vi "RS232 Read Integer Curve Name Replace.vi"(8 "Hardware in":string, 9 "Step Setup in":string, 10 "Setup in":T1={"No.VI"=0, "Category"="", "StepName"="", "Seq setup flattened"="", "Comment"="", "Steps config."=[], "Jump config"=[], "Start"=0.0, "Increment"=0.0, "Name"="Pa", "Unit"="Pa", "Y data"=1, "Y prefix"="", "Y dB ref"=1.0, "Y unit"="", "Repeat State Array"=[]} {"Repeat State Array"."Start" format="%#_5g"; "Y dB ref" format="%.1f"; "Y data" items=["dB", "Lin"]; "Start" format="%#_5g"}, 11 "Type In":string) -> (3 "Inserted Names Out":string[](array[string]))   [LabVIEW 2013]
uses:
  CRYCustom and Run Seq.llb/CRYStep.ctl
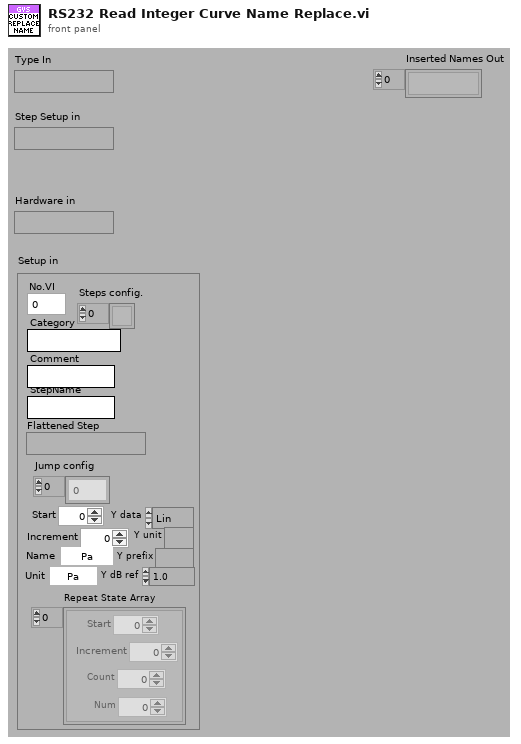
[diagram p1: front panel]
types:
  T1 = typedef "CRYStep.ctl" = cluster{"No.VI":i32, "Category":string, "StepName":string, "Seq setup flattened":string, "Comment":string, "Steps config.":bool[], "Jump config":i32[], "Start":dbl, "Increment":dbl, "Name":string, "Unit":string, "Y data":u16, "Y prefix":string, "Y dB ref":dbl, "Y unit":string, "Repeat State Array":cluster{"Start":dbl, "Increment":dbl, "Count":i32, "Num":i32}[]}
  T2 = cluster{"Type":u16, "Select COM Port":i32, "Byte":i32, "Unit":string, "Curve Name":string}
  T3 = typedef "CRYCustom Cluster.ctl" = cluster{"Help":string, "Flatten Data":string}
  T4 = typedef "CRYData Cluster.ctl" = cluster{"Name":string, "Curve":cluster{"x":dbl, "y":dbl, "z":dbl}[], "X data":u16, "Y data":u16, "Z data":u16, "X axis":u16, "Y axis":u16, "Z axis":u16, "X unit":string, "Y unit":string, "Z unit":string, "X dB ref":dbl, "Y dB ref":dbl, "Z dB ref":dbl, "single val":bool, "protected":bool, "display X":bool, "display Y":bool, "display Z":bool, "Test Info":string, "Step No.":i32, "Plot Settings":cluster{"Color":u32, "Interpolation":u8, "Point Style":u8, "Line Style":u8, "Point Color":u32, "Line Width":u8, "Bar Plot Style":u8, "Fill To":i16}, "AutoProtect":bool}
  T5 = typedef "CRYWaveform Cluster.ctl" = cluster{"Waveform":cluster{"X0":dbl, "dX":dbl, "Y":sgl[]}, "X data":u16, "Y data":u16, "Y axis":u16, "X unit":string, "Y unit":string, "Y dB ref":dbl, "display Y":bool, "display X":bool, "Overload?":bool, "Test Info":string, "Step No.":i32, "Name":string, "protected":bool, "Sqc history":string[], "Signal Channel ID":i32, "Plot Settings":cluster{"Color":u32, "Interpolation":u8, "Point Style":u8, "Line Style":u8, "Point Color":u32, "Line Width":u8, "Bar Plot Style":u8, "Fill To":i16}, "AutoProtect":bool}
  T6 = typedef "CRYResult Cluster.ctl" = cluster{"Name":string, "Margin":dbl, "unit":string, "Verdict":bool, "Limit":string, "Max/Min":string, "protected":bool, "Step No.":i32, "Test Info":string, "AutoProtect":bool}
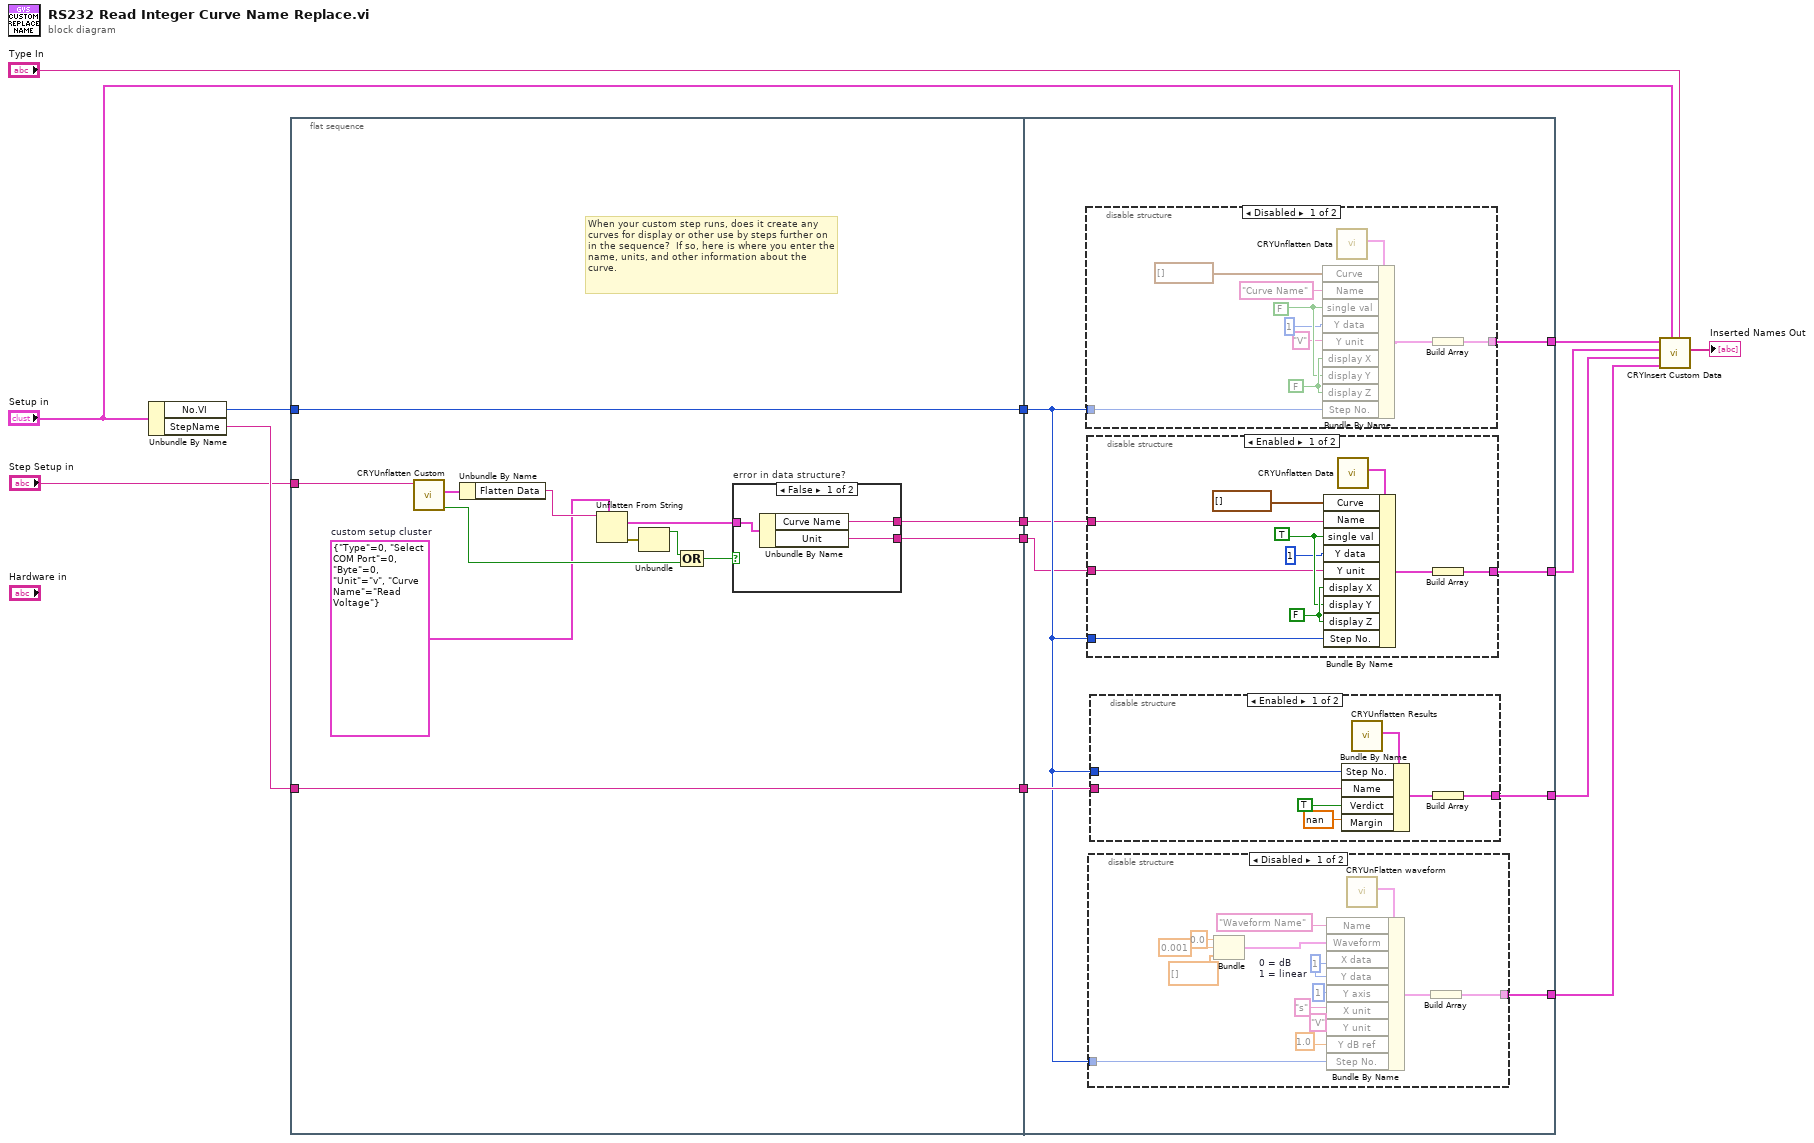
[diagram p0: block diagram]
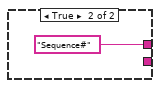
[diagram p2: hidden frame]
diagram:
  n1 = Unbundle By Name("Setup in") -> ("No.VI"=w11:i32, "StepName"=w12:string)
  n2 = flat-sequence {
    tunnel: w11 -> [w26]
    tunnel: w12 -> [w27]
    tunnel: [w27] -> w6
    tunnel: [w26] -> w5
    tunnel: [w21] -> w4
    tunnel: "Step Setup in" -> [w16]
    tunnel: [w15] -> w1
    tunnel: [w37] -> w10
    tunnel: [w36] -> w8
    tunnel: [w35] -> w7
    tunnel: [w34] -> w9
    tunnel: w6 -> [w39]
    tunnel: w5 -> [w38]
    tunnel: w4 -> [w33]
    tunnel: w1 -> [w32]
    frame #0 {
      w17 = T2 {"Type"=0, "Select COM Port"=0, "Byte"=0, "Unit"="v", "Curve Name"="Read Voltage"}  # custom setup cluster
      # "When your custom step runs, does it create any curves for display or other use by steps further on in the sequence?  If so, here is where you enter the name, units, and other information about the curve."
      n3 = call "CRYUnflatten Custom.vi"("Unflatten Custom"=w16) -> ("Error?"=w18:bool, "Custom"=w20:T3)  [unwired: 8 in, 1 out]
      n4 = Unbundle By Name(w20) -> ("Flatten Data"=w19:string)
      n5 = Unflatten From String(type=w17, binary string=w19) -> (value=w24:T2, error out=w25:errorcluster)  [unwired: 1 in, 3 out]
      n6 = Unbundle(w25) -> ("status"=w22:bool)  [unwired: 2 out]
      n7 = Compound Arithmetic op=OR(w22, w18) -> (w23:bool)
      n8 = case "error in data structure?" shown="False" w23 {
        tunnel: w24 -> [w30 _]
        tunnel: [w29 "Sequence#" ("Name")] -> w21
        tunnel: [w28 _] -> w15
        frame False {
          n9 = Unbundle By Name(w30) -> ("Curve Name"=w29:string, "Unit"=w28:string)
        }
        frame True {
        }
      }
    }
    frame #1 {
      n10 = disable-structure shown="Disabled" {
        disable-tunnel: w38 -> [w45 _]
        disable-tunnel: [w40 _] -> w37
        frame Disabled {
          w48 = FALSE
          w47 = FALSE
          n11 = call "CRYUnflatten Data.vi"() -> ("Datum"=w49:T4)  [unwired: 9 in, 2 out]
          n12 = Bundle By Name(cluster=w49, "Curve"=cluster{"x":dbl, "y":dbl, "z":dbl}[] [] ("appended array"), "Name"="Curve Name", "single val"=w47, "Y data"=u16 1, "Y unit"="V", "display X"=w48, "display Y"=w47, "display Z"=w48, "Step No."=w45) -> (w41:T4)
          n13 = Build Array(w41) -> (w40:T4[])
        }
        frame Enabled {
        }
      }
      n14 = disable-structure shown="Enabled" {
        disable-tunnel: w38 -> [w55 _]
        disable-tunnel: w33 -> [w54 _]
        disable-tunnel: [w52 _] -> w34
        disable-tunnel: w32 -> [w50 _]
        frame Enabled {
          w58 = FALSE
          w57 = TRUE
          n15 = call "CRYUnflatten Data.vi"() -> ("Datum"=w59:T4)  [unwired: 9 in, 2 out]
          n16 = Bundle By Name(cluster=w59, "Curve"=cluster{"x":dbl, "y":dbl, "z":dbl}[] [] ("appended array"), "Name"=w54, "single val"=w57, "Y data"=u16 1, "Y unit"=w50, "display X"=w58, "display Y"=w57, "display Z"=w58, "Step No."=w55) -> (w53:T4)
          n17 = Build Array(w53) -> (w52:T4[])
        }
        frame Disabled {
        }
      }
      n18 = disable-structure shown="Disabled" {
        disable-tunnel: [w68 _] -> w35
        disable-tunnel: w38 -> [w67 _]
        frame Disabled {
          w73 = u16 1  # 0 = dB 1 = linear
          n19 = Bundle ("Actual waveform data bundle.\nX0\ndX\n[Y] array")(0.0, 0.001, dbl[] []) -> (w77:cluster{dbl, dbl, dbl[]})  [unwired: 1 out]
          n20 = call "CRYUnFlatten waveform.vi"() -> ("Waveform Cluster"=w78:T5)  [unwired: 9 in, 2 out]
          n21 = Bundle By Name(cluster=w78, "Name"="Waveform Name" ("Bundle Element"), "Waveform"=w77, "X data"=w73, "Y data"=w73, "Y axis"=u16 1, "X unit"="s", "Y unit"="V", "Y dB ref"=1.0, "Step No."=w67) -> (w79:T5)
          n22 = Build Array(w79) -> (w68:T5[])
        }
        frame Enabled {
        }
      }
      n23 = disable-structure shown="Enabled" {
        disable-tunnel: w38 -> [w62 _]
        disable-tunnel: w39 -> [w61 _]
        disable-tunnel: [w60 _] -> w36
        frame Enabled {
          n24 = call "CRYUnflatten Results.vi"() -> ("Result"=w63:T6)  [unwired: 9 in, 2 out]
          n25 = Bundle By Name(cluster=w63, "Step No."=w62, "Name"=w61, "Verdict"=TRUE, "Margin"=nan) -> (w65:T6)
          n26 = Build Array(w65) -> (w60:T6[])
        }
        frame Disabled {
        }
      }
    }
  }
  n27 = call "CRYInsert Custom Data.vi"("sAction"="Type In", "Setup in"="Setup in", "Wave"=w7, "Results"=w8, "Values"=w9, "Curves"=w10) -> ("Inserted Names Out"=→"Inserted Names Out":string[])  [unwired: 4 in, 1 out]
